vi "Xbox Conversion.vi"(2 "Buttons":bool[](array[boolean]), 3 "Axes":dbl[](array[numeric])) -> (0 "Xbox Values":T1)   [LabVIEW 2014]
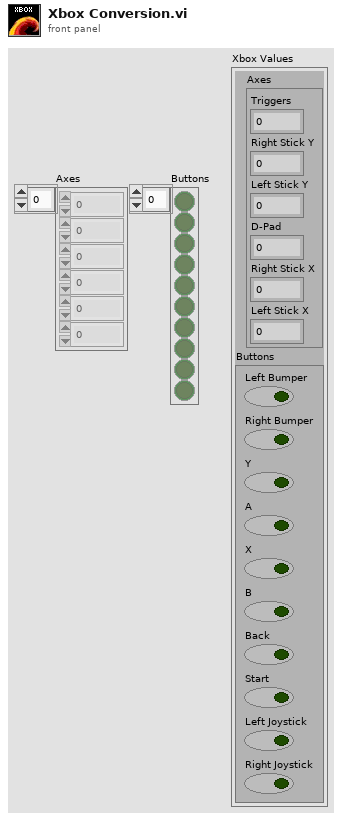
[diagram p1: front panel]
types:
  T1 = cluster{"Axes":cluster{"Triggers":dbl, "Right Stick Y":dbl, "Left Stick Y":dbl, "D-Pad":dbl, "Right Stick X":dbl, "Left Stick X":dbl}, "Buttons":cluster{"Left Bumper":bool, "Right Bumper":bool, "Y":bool, "A":bool, "X":bool, "B":bool, "Back":bool, "Start":bool, "Left Joystick":bool, "Right Joystick":bool}}
  T2 = cluster{"Triggers":dbl, "Right Stick Y":dbl, "Left Stick Y":dbl, "D-Pad":dbl, "Right Stick X":dbl, "Left Stick X":dbl}
  T3 = cluster{"Left Bumper":bool, "Right Bumper":bool, "Y":bool, "A":bool, "X":bool, "B":bool, "Back":bool, "Start":bool, "Left Joystick":bool, "Right Joystick":bool}
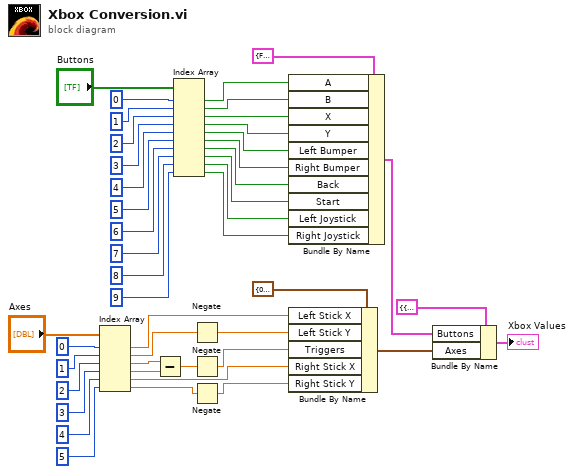
[diagram p0: block diagram]
diagram:
  n1 = Index Array(array="Axes", index #1=0 ("index"), index #2=1 ("index"), index #3=2 ("index"), index #4=3 ("index"), index #5=4 ("index"), index #6=5 ("index")) -> (element #1=w27:dbl, element #2=w26:dbl, element #3=w25:dbl, element #4=w24:dbl, element #5=w22:dbl, element #6=w21:dbl)
  n2 = Subtract(x=w25, y=w24) -> (x-y=w23:dbl)
  n3 = Index Array(array="Buttons", index #1=0 ("index"), index #2=1 ("index"), index #3=2 ("index"), index #4=3 ("index"), index #5=4 ("index"), index #6=5 ("index"), index #7=6 ("index"), index #8=7 ("index"), index #9=8 ("index"), index #10=9 ("index")) -> (element #1=w10:bool, element #2=w9:bool, element #3=w8:bool, element #4=w7:bool, element #5=w6:bool, element #6=w5:bool, element #7=w4:bool, element #8=w3:bool, element #9=w2:bool, element #10=w1:bool)
  n4 = Negate(x=w26) -> (-x=w38:dbl)
  n5 = Negate(x=w23) -> (-x=w37:dbl)
  n6 = Negate(x=w21) -> (-x=w36:dbl)
  n7 = Bundle By Name(cluster=T3 {"Left Bumper"=FALSE, "Right Bumper"=FALSE, "Y"=FALSE, "A"=FALSE, "X"=FALSE, "B"=FALSE, "Back"=FALSE, "Start"=FALSE, "Left Joystick"=FALSE, "Right Joystick"=FALSE}, "A"=w10, "B"=w9, "X"=w8, "Y"=w7, "Left Bumper"=w6, "Right Bumper"=w5, "Back"=w4, "Start"=w3, "Left Joystick"=w2, "Right Joystick"=w1) -> (w41:T3)
  n8 = Bundle By Name(cluster=T2 {"Triggers"=0.0, "Right Stick Y"=0.0, "Left Stick Y"=0.0, "D-Pad"=0.0, "Right Stick X"=0.0, "Left Stick X"=0.0}, "Left Stick X"=w27, "Left Stick Y"=w38, "Triggers"=w37, "Right Stick X"=w22, "Right Stick Y"=w36) -> (w40:T2)
  n9 = Bundle By Name(cluster=T1 {"Axes"={"Triggers"=0.0, "Right Stick Y"=0.0, "Left Stick Y"=0.0, "D-Pad"=0.0, "Right Stick X"=0.0, "Left Stick X"=0.0}, "Buttons"={"Left Bumper"=FALSE, "Right Bumper"=FALSE, "Y"=FALSE, "A"=FALSE, "X"=FALSE, "B"=FALSE, "Back"=FALSE, "Start"=FALSE, "Left Joystick"=FALSE, "Right Joystick"=FALSE}}, "Buttons"=w41, "Axes"=w40) -> (→"Xbox Values":T1)
